vi "NavX Data Processing.vi"(10 "State In":enum16{"Reset", "Collect Data"}(ring), 11 "Cluster":T16 {"navX Device"."Interface"."Update Rate (4Hz-60Hz)" min=4 max=60 step=1; "SonarMB1010AnalogDevRef"."Average Bits" max=15}) -> (2 "State Out":enum16{"Reset", "Collect Data"}(ring))   [LabVIEW 2015]
uses:
  navX Library v2/TypeDefs/Z900_navX_DeviceTypeDef.ctl
  navX Library v2/TypeDefs/Z900_navX_ProtocolTypeDef.ctl
  navX Library v2/TypeDefs/Z900_navX_NotifyPacketTypeDef.ctl
  navX Library v2/TypeDefs/Z900_navX_ActionTypeDef.ctl
  <vilib>/Rock Robotics/WPI/Joystick/WPI_JoystickDevRef.ctl
  <vilib>/Rock Robotics/WPI/Joystick/WPI_JoystickDeviceEnum.ctl
  <vilib>/Rock Robotics/WPI/RobotDrive/WPI_RobotDriveDevRef.ctl
  <vilib>/Rock Robotics/WPI/MotorControl/WPI_MotorControlDeviceRef.ctl
  <vilib>/Rock Robotics/WPI/MotorControl/WPI_MotorControlType.ctl
  <vilib>/Rock Robotics/SystemInterfaces/DIO/FPGA_DIOPWMChannel.ctl
  <vilib>/Rock Robotics/WPI/PWM/WPI_PWMDeadband.ctl
  <vilib>/Rock Robotics/WPI/CAN/Jaguar/SubVIs/WPI_CANJaguar_ControlMode.ctl
  <vilib>/Rock Robotics/WPI/CAN/TalonSRX/WPI_CANTalonSRX_APIControlMode.ctl
  <vilib>/Rock Robotics/WPI/Ultrasonic/WPI_SonarMB1010AnalogDeviceRef.ctl
  <vilib>/Rock Robotics/WPI/AnalogChannel/WPI_AnalogChannelDevRef.ctl
  <vilib>/Rock Robotics/SystemInterfaces/AI/FPGA_AIChannel.ctl
  Robot Global Data.vi
  <vilib>/Rock Robotics/Network Tables/NT Write Numeric Array.vi
  navX Library v2/navX Library v2.lvlib
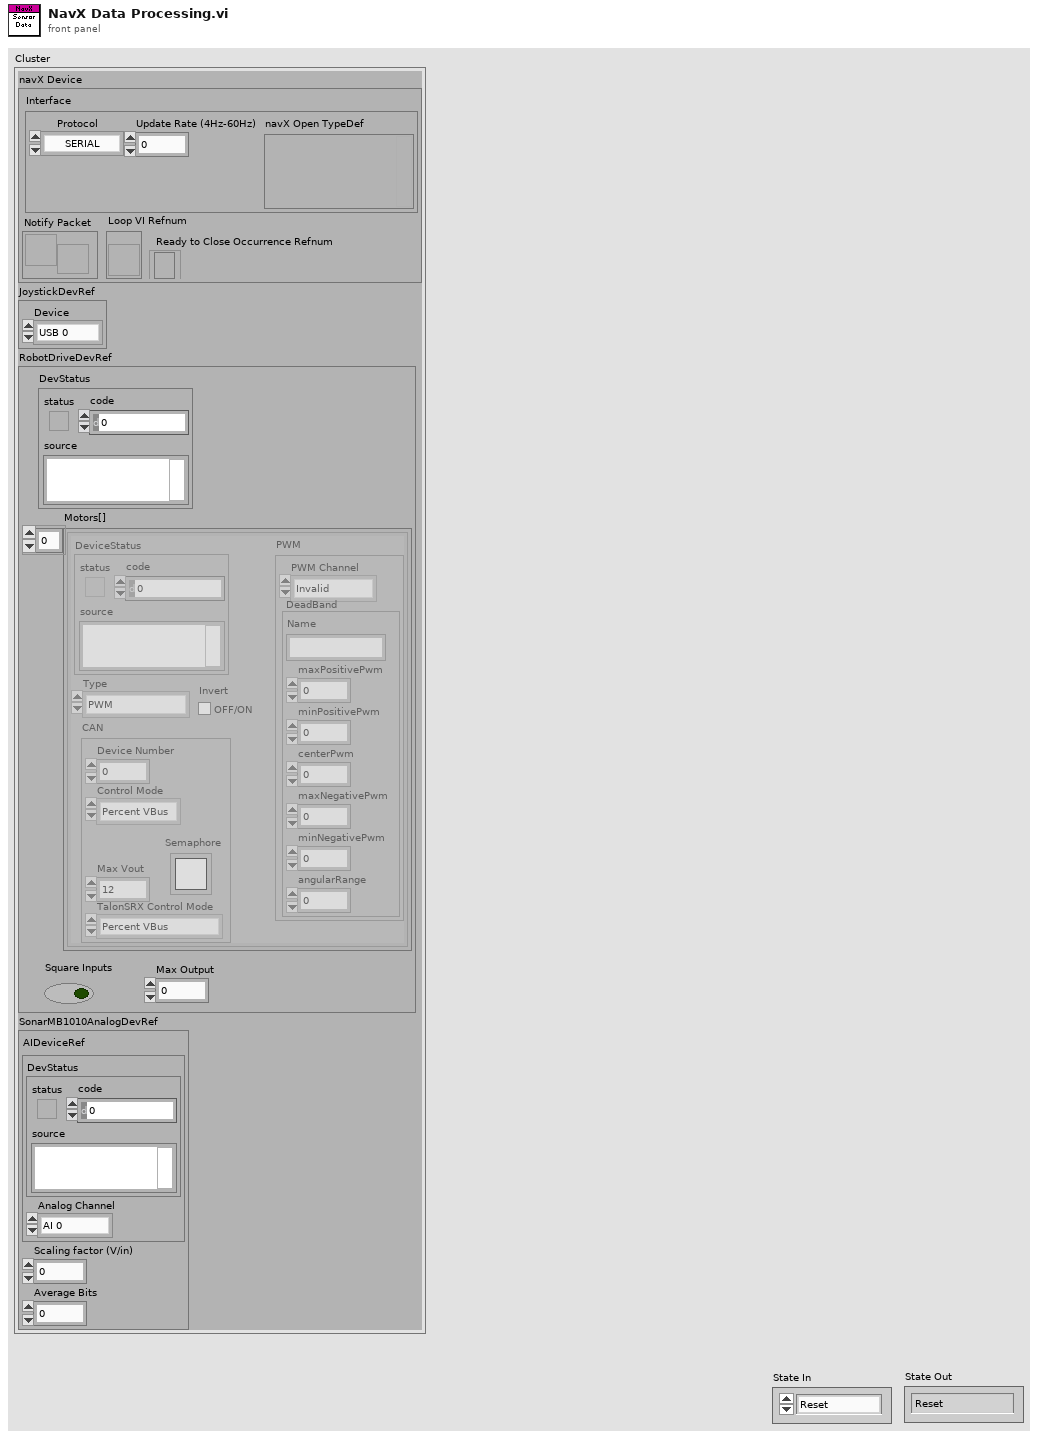
[diagram p1: front panel]
types:
  T1 = typedef "navX Library v2.lvlib/Z900_navX_DeviceTypeDef.ctl" = cluster{"Interface":cluster{"Protocol":T2, "Update Rate (4Hz-60Hz)":u8, "navX Open TypeDef":variant}, "Notify Packet":refnum<notifier>, "Loop VI Refnum":refnum<vi>, "Ready to Close Occurrence Refnum":refnum<k4>}
  T2 = typedef "navX Library v2.lvlib/Z900_navX_ProtocolTypeDef.ctl" = enum16{"SERIAL", "I2C", "SPI"}
  T3 = typedef "WPI_JoystickDevRef.ctl" = cluster{"Device":T4}
  T4 = typedef "WPI_JoystickDeviceEnum.ctl" = enum16{"USB 0", "USB 1", "USB 2", "USB 3", "USB 4", "USB 5"}
  T5 = typedef "WPI_RobotDriveDevRef.ctl" = cluster{"DevStatus":errorcluster, "Motors[]":T6[], "Square Inputs":bool, "Max Output":dbl}
  T6 = typedef "WPI_MotorControlDeviceRef.ctl" = cluster{"DeviceStatus":errorcluster, "Type":T7, "PWM":cluster{"PWM Channel":T8, "DeadBand":T9}, "CAN":cluster{"Device Number":u8, "Control Mode":T10, "Semaphore":T11, "Max Vout":dbl, "TalonSRX Control Mode":T12}, "Invert":bool}
  T7 = typedef "WPI_MotorControlType.ctl" = enum16{"PWM", "CAN", "CANTalonSRX"}
  T8 = typedef "FPGA_DIOPWMChannel.ctl" = enum8{"PWM 0", "PWM 1", "PWM 2", "PWM 3", "PWM 4", "PWM 5", "PWM 6", "PWM 7", "PWM 8", "PWM 9", "PWM MXP 0", "PWM MXP 1", "PWM MXP 2", "PWM MXP 3", "PWM MXP 4", "PWM MXP 5", "PWM MXP 6", "PWM MXP 7", "PWM MXP 8", "PWM MXP 9", "Invalid"}
  T9 = typedef "WPI_PWMDeadband.ctl" = cluster{"Name":string, "maxPositivePwm":i32, "minPositivePwm":i32, "centerPwm":i32, "maxNegativePwm":i32, "minNegativePwm":i32, "angularRange":u16}
  T10 = typedef "WPI_CANJaguar_ControlMode.ctl" = enum8{"Percent VBus", "Current", "Speed", "Position", "Voltage"}
  T11 = typedef "Semaphore RefNum" = refnum<k1>
  T12 = typedef "WPI_CANTalonSRX_APIControlMode.ctl" = enum8{"Percent VBus", "Speed", "Position", "Slave", "Unchanged / Invalid", "Voltage Compensation", "Current", "Motion Profile"}
  T13 = typedef "WPI_SonarMB1010AnalogDeviceRef.ctl" = cluster{"AIDeviceRef":T14, "Scaling factor (V/in)":dbl, "Average Bits":u8}
  T14 = typedef "WPI_AnalogChannelDevRef.ctl" = cluster{"DevStatus":errorcluster, "Analog Channel":T15}
  T15 = typedef "FPGA_AIChannel.ctl" = enum8{"AI 0", "AI 1", "AI 2", "AI 3", "AI MXP 0", "AI MXP 1", "AI MXP 2", "AI MXP 3", "Invalid"}
  T16 = cluster{"navX Device":T1, "JoystickDevRef":T3, "RobotDriveDevRef":T5, "SonarMB1010AnalogDevRef":T13}
  T17 = cluster{"Yaw":dbl, "Roll":dbl, "Pitch":dbl, "Heading":dbl, "Fused Heading":dbl}
  T18 = cluster{"LinearAcceleration X":dbl, "LinearAcceleration Y":dbl, "LinearAcceleration Z":dbl}
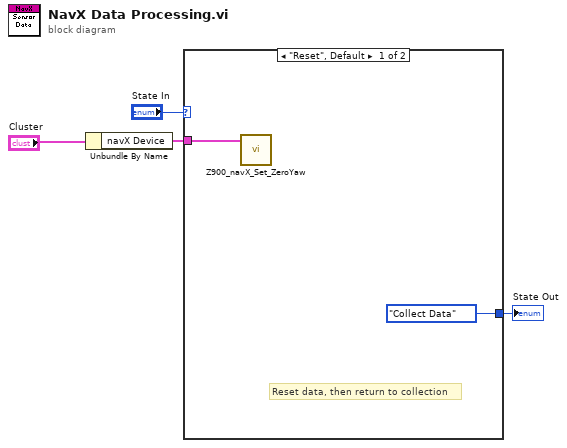
[diagram p0: block diagram]
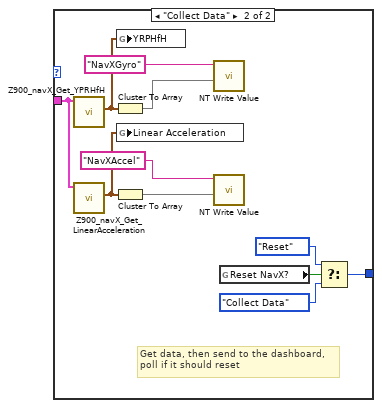
[diagram p2: hidden frame]
diagram:
  n1 = Unbundle By Name("Cluster") -> ("navX Device"=w4:T1)
  n2 = case shown="\"Reset\", Default" "State In" {
    tunnel: w4 -> [w5 w17]
    tunnel: [enum16{"Reset", "Collect Data"}."Collect Data" ("State In") w7] -> w2
    frame "Reset", Default {
      # "Reset data, then return to collection"
      n3 = call "Z900_navX_Set_ZeroYaw.vi"("navX Device"=w5) -> ()  [unwired: 9 in, 2 out]
    }
    frame "Collect Data" {
      # "Get data, then send to the dashboard,\npoll if it should reset"
      n4 = call "Z900_navX_Get_YPRHfH.vi"("navX Device"=w17) -> ("YRPHfH"=w16:T17)  [unwired: 7 in, 3 out]
      n5 = call "Z900_navX_Get_LinearAcceleration.vi"("navX Device"=w17) -> ("Linear Acceleration"=w13:T18)  [unwired: 7 in, 3 out]
      n6 = Cluster To Array(cluster=w16) -> (array=w15:dbl[])
      n7 = Cluster To Array(cluster=w13) -> (array=w11:dbl[])
      n8 = global write "Robot Global Data.vi" "YRPHfH"(w16) -> ()
      n9 = global write "Robot Global Data.vi" "Linear Acceleration"(w13) -> ()
      n10 = call-poly <vilib>:"NT Write Value.vi"("Numeric Array"=w15, "Name"="NavXGyro") -> ()  [unwired: 9 in, 1 out]
      n11 = call-poly <vilib>:"NT Write Value.vi"("Numeric Array"=w11, "Name"="NavXAccel") -> ()  [unwired: 9 in, 1 out]
      n12 = global read "Robot Global Data.vi" "Reset NavX?"() -> (w10:bool)
      n13 = Select(t=enum16{"Reset", "Collect Data"}."Reset" ("State In"), s=w10, f=enum16{"Reset", "Collect Data"}."Collect Data" ("State In")) -> (s? t:f=w7:enum16{"Reset", "Collect Data"})
    }
  }
  "State Out" <- w2
